vi "Parametric Calculations.vi"(0 "Data Management Control":T1, 2 "Specific Voltages":dbl[](array[numeric])=[32.0, 36.0], 5 "Selected Exp Settings":T2={"P2_Sweep_Stop_V"=36.0, "P2_Sweep_Step_V"=1.0, "Experiment Name"="", "Resistance Threshold"=1.0, "P1_Fixed_Voltage"=36.0, "P2_Sweep_Start_V"=36.0}, 13 "Cal Measurements":T3 {"Port 3 Capacitance" format="%#_6p"; "Port 2 Capacitance" format="%#_6p"; "Port 1 Capacitance" format="%#_6p"}) -> (4 "Parametric Calculated Values":T4={"Voltage Calculated Values"={"P1_VPD_C"=0.0, "P2_VPD_C"=0.0, "P1_VPD_Rel_C"=0.0, "P2_VPD_Rel_C"=0.0}, "Resistance Calculated Values"={"Rc_free"=0.0, "Rc_first"=0.0, "Rc_vmax"=0.0, "Rc_last"=0.0, "Rc_end"=0.0, "VPD_R"=0.0, "VPD_Rel_R"=0.0}, "Capacitance Calculated Values"={"P1_CPD_free"=0.0, "P2_CPD_free"=0.0, "P1_CPD_vmax"=0.0, "P2_CPD_vmax"=0.0, "P1_CPD_first"=0.0, "P2_CPD_first"=0.0, "P1_CPD_last"=0.0, "P2_CPD_last"=0.0, "P1_CPD_end"=0.0, "P2_CPD_end"=0.0, "P1_CPD_max"=0.0, "P2_CPD_max "=0.0, "CPD_Free"=0.0, "CPD_First"=0.0, "CPD_max"=0.0, "CPD_Last"=0.0, "CPD_End"=0.0, "CPD_vmax"=0.0}, "Cap Calc Arrays"={"CPD_sum"=[], "P2_CPD@V"=[], "P1_CPD@V"=[], "Specific Voltages"=[32.0, 36.0]}, "Resistance Array Calc"={"RC@V"=[]}, "TN4 Calc"={"P1_TN4_ACT"=0.0, "P2_TN4_ACT "=0.0, "VPD_R_2"=0.0, "DVR"=0.0}, "Corrected_Capacitance Calculated Values"={"P1_CPD_free"=0.0, "P2_CPD_free"=0.0, "P1_CPD_vmax"=0.0, "P2_CPD_vmax"=0.0, "P1_CPD_first"=0.0, "P2_CPD_first"=0.0, "P1_CPD_last"=0.0, "P2_CPD_last"=0.0, "P1_CPD_end"=0.0, "P2_CPD_end"=0.0, "P1_CPD_max"=0.0, "P2_CPD_max "=0.0, "CPD_Free"=0.0, "CPD_First"=0.0, "CPD_max"=0.0, "CPD_Last"=0.0, "CPD_End"=0.0, "CPD_vmax"=0.0}})   [LabVIEW 2013]
uses:
  Controls/Data Management.ctl
  Controls/Individual User Inputs.ctl
  Controls/Parametric Calculated Values.ctl
  Controls/Voltage Calculated Values.ctl
  Controls/Resistance Individual Calculated Values.ctl
  Controls/Capacitance Individual Calculated Values.ctl
  Controls/Capacitance Array Calculated Values.ctl
  Controls/Resistance Array Calculated Values.ctl
  Controls/TN4 Calc.ctl
  Controls/Corrected_Capacitance Individual Calculated Values.ctl
  Controls/ENA_Marker Measurements.ctl
panel:
  out "Error Out":errorcluster
  in  "Error In":errorcluster
  in  "Tab Control":enum32{"Inputs", "Outputs"}(tab)
  # "Test Settings"
  # "Make the Stop and Step Negative \nfor negative sweep"
  # "Calculation Settings"
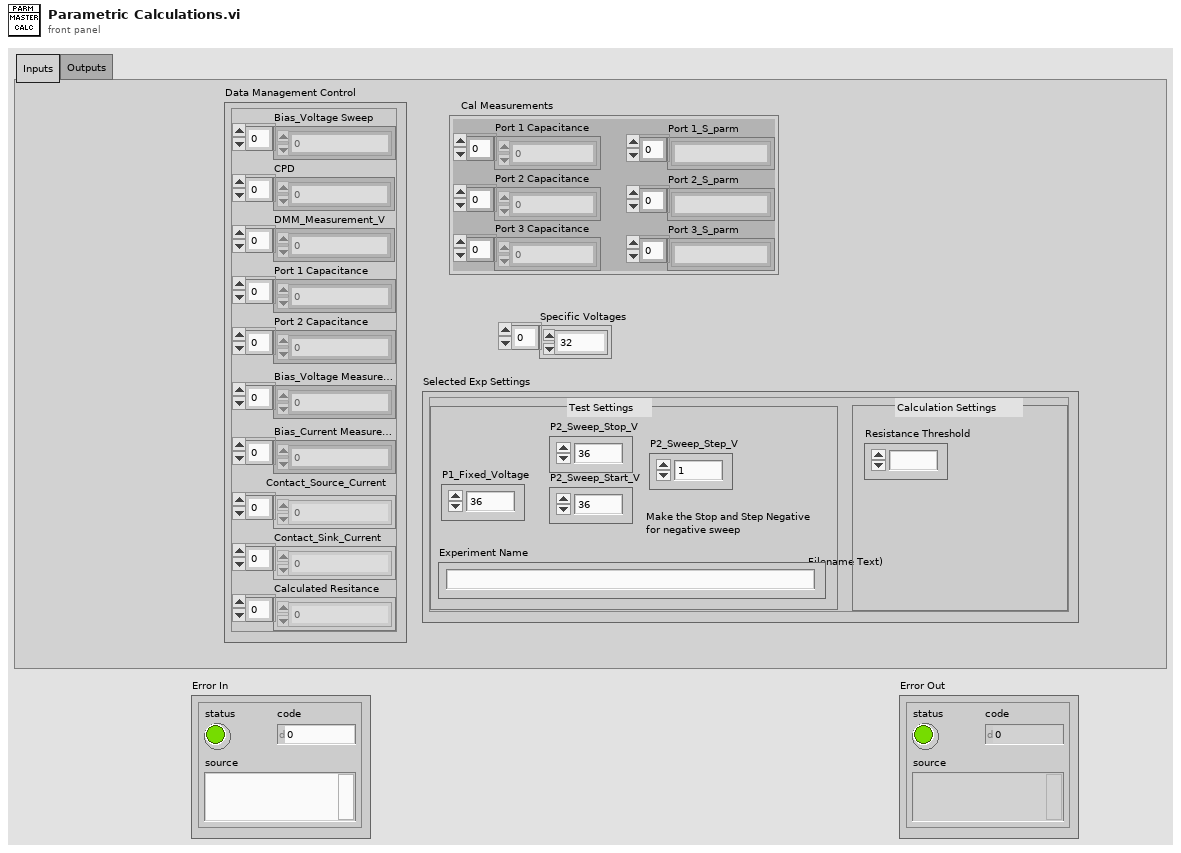
[diagram p1: front panel]
types:
  T1 = typedef "Data Management.ctl" = cluster{"Bias_Voltage Sweep":dbl[], "CPD":dbl[], "DMM_Measurement_V":dbl[], "Port 1 Capacitance":dbl[], "Port 2 Capacitance":dbl[], "Bias_Voltage Measurement":dbl[], "Bias_Current Measurement":dbl[], "Contact_Source_Current":dbl[], "Contact_Sink_Current":dbl[], "Calculated Resitance":dbl[]}
  T2 = typedef "Individual User Inputs.ctl" = cluster{"P2_Sweep_Stop_V":dbl, "P2_Sweep_Step_V":dbl, "Experiment Name":string, "Resistance Threshold":dbl, "P1_Fixed_Voltage":dbl, "P2_Sweep_Start_V":dbl}
  T3 = typedef "ENA_Marker Measurements.ctl" = cluster{"Port 1 Capacitance":dbl[], "Port 2 Capacitance":dbl[], "Port 3 Capacitance":dbl[], "Port 1_S_parm":string[], "Port 2_S_parm":string[], "Port 3_S_parm":string[]}
  T4 = typedef "Parametric Calculated Values.ctl" = cluster{"Voltage Calculated Values":T5, "Resistance Calculated Values":T6, "Capacitance Calculated Values":T7, "Cap Calc Arrays":T8, "Resistance Array Calc":T9, "TN4 Calc":T10, "Corrected_Capacitance Calculated Values":T11}
  T5 = typedef "Voltage Calculated Values.ctl" = cluster{"P1_VPD_C":dbl, "P2_VPD_C":dbl, "P1_VPD_Rel_C":dbl, "P2_VPD_Rel_C":dbl}
  T6 = typedef "Resistance Individual Calculated Values.ctl" = cluster{"Rc_free":dbl, "Rc_first":dbl, "Rc_vmax":dbl, "Rc_last":dbl, "Rc_end":dbl, "VPD_R":dbl, "VPD_Rel_R":dbl}
  T7 = typedef "Capacitance Individual Calculated Values.ctl" = cluster{"P1_CPD_free":dbl, "P2_CPD_free":dbl, "P1_CPD_vmax":dbl, "P2_CPD_vmax":dbl, "P1_CPD_first":dbl, "P2_CPD_first":dbl, "P1_CPD_last":dbl, "P2_CPD_last":dbl, "P1_CPD_end":dbl, "P2_CPD_end":dbl, "P1_CPD_max":dbl, "P2_CPD_max ":dbl, "CPD_Free":dbl, "CPD_First":dbl, "CPD_max":dbl, "CPD_Last":dbl, "CPD_End":dbl, "CPD_vmax":dbl}
  T8 = typedef "Capacitance Array Calculated Values.ctl" = cluster{"CPD_sum":dbl[], "P2_CPD@V":dbl[], "P1_CPD@V":dbl[], "Specific Voltages":dbl[]}
  T9 = typedef "Resistance Array Calculated Values.ctl" = cluster{"RC@V":dbl[]}
  T10 = typedef "TN4 Calc.ctl" = cluster{"P1_TN4_ACT":dbl, "P2_TN4_ACT ":dbl, "VPD_R_2":dbl, "DVR":dbl}
  T11 = typedef "Corrected_Capacitance Individual Calculated Values.ctl" = cluster{"P1_CPD_free":dbl, "P2_CPD_free":dbl, "P1_CPD_vmax":dbl, "P2_CPD_vmax":dbl, "P1_CPD_first":dbl, "P2_CPD_first":dbl, "P1_CPD_last":dbl, "P2_CPD_last":dbl, "P1_CPD_end":dbl, "P2_CPD_end":dbl, "P1_CPD_max":dbl, "P2_CPD_max ":dbl, "CPD_Free":dbl, "CPD_First":dbl, "CPD_max":dbl, "CPD_Last":dbl, "CPD_End":dbl, "CPD_vmax":dbl}
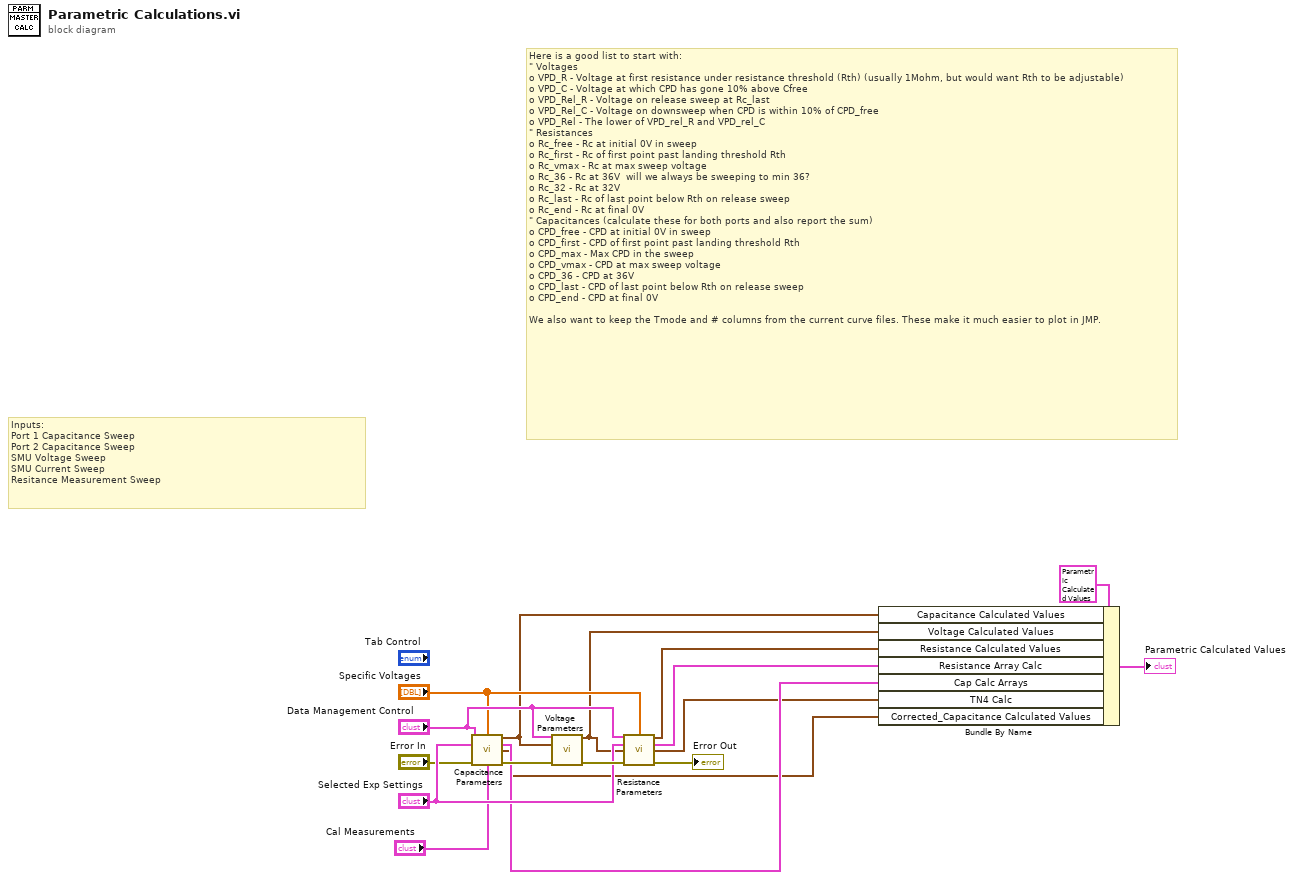
[diagram p0: block diagram]
diagram:
  # "Inputs:\nPort 1 Capacitance Sweep\nPort 2 Capacitance Sweep\nSMU Voltage Sweep\nSMU Current Sweep\nResitance Measurement Sweep"
  # "Here is a good list to start with:\n\"\tVoltages\no\tVPD_R - Voltage at first resistance under resistance threshold (Rth) (usually 1Mohm, but would want Rth to be adjustable)\no\tVPD_C - Voltage at which CPD has gone 10% above Cfree\no\tVPD_Rel_R - Voltage on release sweep at Rc_last\no\tVPD_Rel_C - Voltage on downsweep when CPD is within 10% of CPD_free\no\tVPD_Rel - The lower of VPD_rel_R and VPD_rel_C\n\"\tResistances\no\tRc_free - Rc at initial 0V in sweep\no\tRc_first - Rc of first point past landing threshold Rth \no\tRc_vmax - Rc at max sweep voltage\no\tRc_36 - Rc at 36V  will we always be sweeping to min 36?\no\tRc_32 - Rc at 32V\no\tRc_last - Rc of last point below Rth on release sweep\no\tRc_end - Rc at final 0V\n\"\tCapacitances (calculate these for both ports and also report the sum)\no\tCPD_free - CPD at initial 0V in sweep\no\tCPD_first - CPD of first point past landing threshold Rth \no\tCPD_max - Max CPD in the sweep\no\tCPD_vmax - CPD at max sweep voltage\no\tCPD_36 - CPD at 36V\no\tCPD_last - CPD of last point below Rth on release sweep\no\tCPD_end - CPD at final 0V\n \nWe also want to keep the Tmode and # columns from the current curve files. These make it much easier to plot in JMP."
  n1 = call "Capacitance Parameters.vi"("Data Management Control"="Data Management Control", "Specific Voltages"="Specific Voltages", "Selected Exp Settings"="Selected Exp Settings", "Error In"="Error In", "Cal Measurements"="Cal Measurements") -> ("Capacitance Calculated Values"=w10:T7, "Cap Calc Arrays"=w6:T8, "Corrected_Capacitance Calculated Values"=w1:T11, "Error Out"=w16:errorcluster)  [unwired: 7 in]
  n2 = call "Voltage Parameters.vi"("Data Management Control"="Data Management Control", "Capacitance Calculated Values"=w10, "Error In"=w16) -> ("Voltage Calculated Values"=w4:T5, "Error Out"=w15:errorcluster)  [unwired: 11 in]
  n3 = call "Resistance Parameters.vi"("Data Management Control"="Data Management Control", "Specific Voltages 2"="Specific Voltages", "Selected Exp Settings"="Selected Exp Settings", "Voltage Calculated Values"=w4, "Error In"=w15) -> ("Resistance Calculated Values"=w5:T6, "Resistance Array Calc"=w7:T9, "TN4 Calc"=w3:T10, "Error Out"=→"Error Out":errorcluster)  [unwired: 7 in]
  n4 = Bundle By Name(cluster=T4 {"Voltage Calculated Values"={"P1_VPD_C"=0.0, "P2_VPD_C"=0.0, "P1_VPD_Rel_C"=0.0, "P2_VPD_Rel_C"=0.0}, "Resistance Calculated Values"={"Rc_free"=0.0, "Rc_first"=0.0, "Rc_vmax"=0.0, "Rc_last"=0.0, "Rc_end"=0.0, "VPD_R"=0.0, "VPD_Rel_R"=0.0}, "Capacitance Calculated Values"={"P1_CPD_free"=0.0, "P2_CPD_free"=0.0, "P1_CPD_vmax"=0.0, "P2_CPD_vmax"=0.0, "P1_CPD_first"=0.0, "P2_CPD_first"=0.0, "P1_CPD_last"=0.0, "P2_CPD_last"=0.0, "P1_CPD_end"=0.0, "P2_CPD_end"=0.0, "P1_CPD_max"=0.0, "P2_CPD_max "=0.0, "CPD_Free"=0.0, "CPD_First"=0.0, "CPD_max"=0.0, "CPD_Last"=0.0, "CPD_End"=0.0, "CPD_vmax"=0.0}, "Cap Calc Arrays"={"CPD_sum"=[], "P2_CPD@V"=[], "P1_CPD@V"=[], "Specific Voltages"=[]}, "Resistance Array Calc"={"RC@V"=[]}, "TN4 Calc"={"P1_TN4_ACT"=0.0, "P2_TN4_ACT "=0.0, "VPD_R_2"=0.0, "DVR"=0.0}, "Corrected_Capacitance Calculated Values"={"P1_CPD_free"=0.0, "P2_CPD_free"=0.0, "P1_CPD_vmax"=0.0, "P2_CPD_vmax"=0.0, "P1_CPD_first"=0.0, "P2_CPD_first"=0.0, "P1_CPD_last"=0.0, "P2_CPD_last"=0.0, "P1_CPD_end"=0.0, "P2_CPD_end"=0.0, "P1_CPD_max"=0.0, "P2_CPD_max "=0.0, "CPD_Free"=0.0, "CPD_First"=0.0, "CPD_max"=0.0, "CPD_Last"=0.0, "CPD_End"=0.0, "CPD_vmax"=0.0}} ("Parametric Calculated Values 2"), "Capacitance Calculated Values"=w10, "Voltage Calculated Values"=w4, "Resistance Calculated Values"=w5, "Resistance Array Calc"=w7, "Cap Calc Arrays"=w6, "TN4 Calc"=w3, "Corrected_Capacitance Calculated Values"=w1) -> (→"Parametric Calculated Values":T4)
